vi "KeyInput.vi"() -> ()   [LabVIEW 2021]
uses:
  <vilib>/event_ctls.llb/eventvkey.ctl
panel:
  out "InputDetect":string
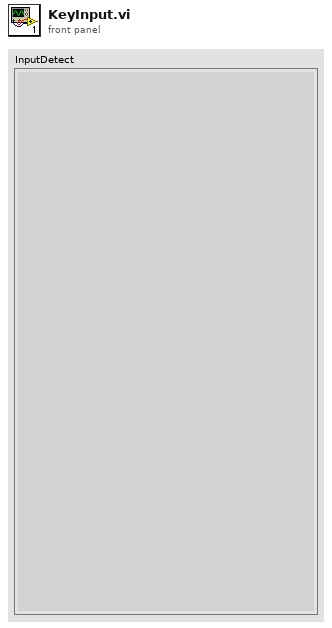
[diagram p1: front panel]
types:
  T1 = typedef "eventvkey.ctl" = enum16{"ASCII", "Enter", "Return", "Shift", "Ctrl", "Alt", "Cmd", "Opt", "Caps", "NumLock", "Clear", "Break", "Up", "Down", "Left", "Right", "Insert", "Delete", "Home", "End", "PageUp", "PageDown", "Escape", "Help", "Pause", "ScrollLock", "F1", "F2", "F3", "F4", "F5", "F6", "F7", "F8", "F9", "F10", "F11", "F12", "F13", "F14", "F15", "F16", "F17", "F18", "F19", "F20", "F21", "F22", "F23", "F24", "Play", "VolumeUp", "VolumeDown", "Mute", "Two Byte Char"}
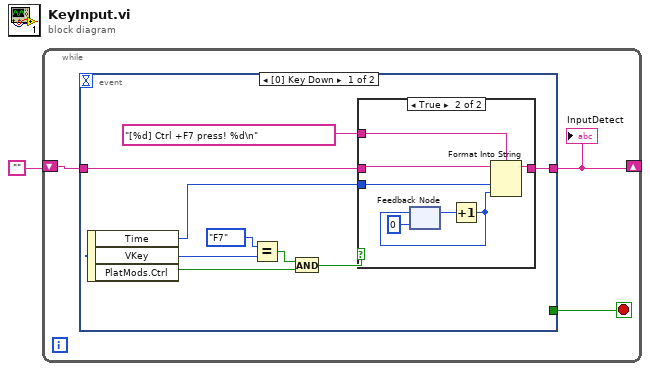
[diagram p0: block diagram]
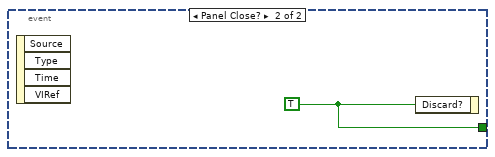
[diagram p3: hidden frame]
diagram:
  n1 = while {
    shift-right: [w3] -> _
    shift-left: "" -> [w2]
    stop <- w4 stop-if-true
    n2 = event shown="[0] Key Down" {
      selector: _ -> [_ _]
      dyn-events: _ -> [_ _]
      timeout: _ -> [_ _]
      tunnel: [_ w22] -> w4
      tunnel: [w8 _] -> w3
      tunnel: w2 -> [w7 _]
      event Key Down {
        n3 = event-data() -> ("Time"=w6:u32, "VKey"=w13:T1, "PlatMods.Ctrl"=w10:bool)  [unwired: 1 in]
        n4 = Equal?(x=eventvkey."F7" ("VKey"), y=w13) -> (x = y?=w11:bool)
        n5 = And(x=w11, y=w10) -> (x .and. y?=w9:bool)
        n6 = case shown="True" w9 {
          tunnel: [w14 w20] -> w8
          tunnel: w7 -> [w14 w21]
          tunnel: w6 -> [_ w19]
          tunnel: "[%d] Ctrl +F7 press! %d\n" ("format string") -> [_ w18]
          frame False {
          }
          frame True {
            n7 = feedback #1(0) -> (w16:i32)
            n8 = Increment(x=w16) -> (x+1=w15:i32)
            n9 = feedback-in #1(w15) -> ()
            n10 = Format Into String(format string=w18, initial string=w21, w19, w15) -> (resulting string=w20:string)  [unwired: 1 in, 1 out]
          }
        }
      }
      event Panel Close? {
        w22 = TRUE ("Discard?")
        n11 = event-data() -> ()  [unwired: 1 in, 4 out]
        n12 = event-data("Discard?"=w22) -> ()  [unwired: 1 in, 1 out]
      }
    }
    "InputDetect" <- w3
  }
